vi "Exercise 4.3 Webcam to JPG.vi"() -> ()   [LabVIEW 2014]
uses:
  <vilib>/Q-Wave Systems/QwaveSys RPi Training Package (Demo)/Addons/QwaveSys RPi Training Library.lvlib
panel:
  out "Output 2":picture
  out "string":string
  in  "file path":path=path "/home/pi/temp.jpg"
  out "Output":picture
  in  "Image Size":T1(ring)
  in  "camnum":i32
  out "return type":i32
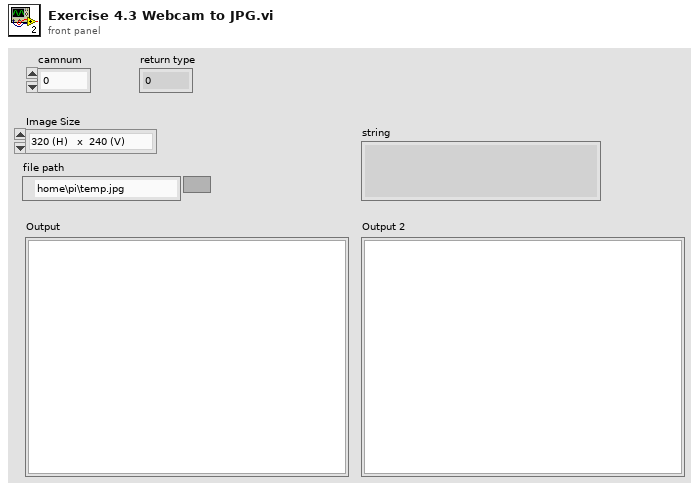
[diagram p1: front panel]
types:
  T1 = enum16{"320 (H)   x  240 (V)", "352(H)    x  288 (V)", "640 (H)   x  480 (V) ", "800 (H)   x  600 (V)", "1024 (H) x  768 (V)", "1280 (H) x  720 (V)", "1280 (H) x 1024 (V)", "1920 (H) x 1080 (V)"}
  T2 = typedef "imagedata.ctl" = cluster{"image type":i32, "image depth":i32, "image":u8[], "mask":u8[], "colors":u32[], "Rectangle":cluster{"left":i16, "top":i16, "right":i16, "bottom":i16}}
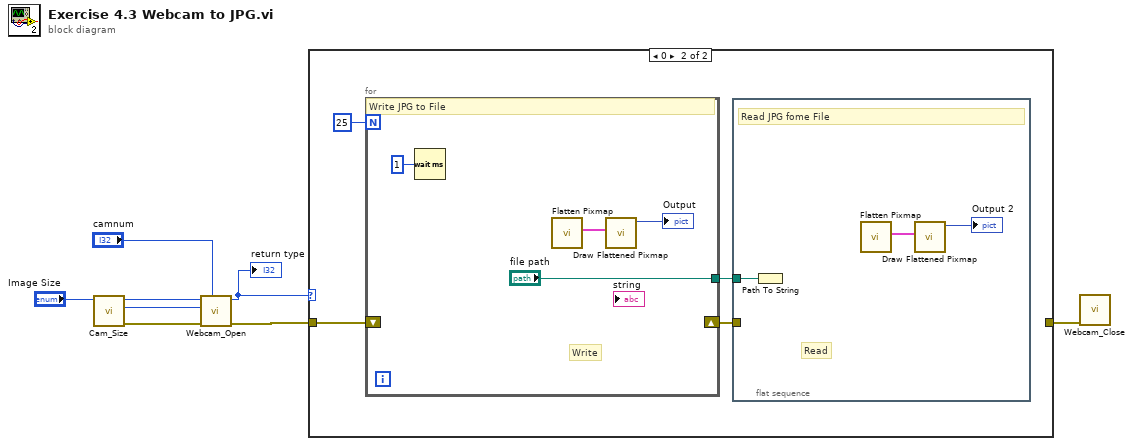
[diagram p0: block diagram]
diagram:
  n1 = call <vilib>:"Cam_Size.vi"("Image Size"="Image Size") -> ("error out"=w7:errorcluster, "h"=w6:i32, "w"=w5:i32)  [unwired: 8 in]
  n2 = call <vilib>:"Webcam_Open.vi"("webcamnum"="camnum", "error in (no error)"=w7, "height"=w6, "width"=w5) -> ("error out"=w3:errorcluster, "return type"=w2:i32)  [unwired: 6 in]
  "return type" <- w2
  n3 = case shown="0" w2 {
    tunnel: w3 -> [w9 w13]
    tunnel: [w9 _] -> w1
    frame -1, Default {
    }
    frame 0 {
      n4 = for {
        N: 25 -> [_]
        shift-right: [_] -> w10
        shift-left: w13 -> [_]
        tunnel: ["file path"] -> w11
        # "Write"
        # "Write JPG to File"
        n5 = Wait (ms)(milliseconds to wait=u32 1) -> ()  [unwired: 1 out]
        n6 = call <vilib>:"Flatten Pixmap.vi"() -> ("image data"=w19:T2)  [unwired: 11 in]
        n7 = call <vilib>:"Draw Flattened Pixmap.vi"("image data"=w19) -> ("new picture"=→"Output":picture)  [unwired: 8 in]
      }
      n8 = flat-sequence {
        tunnel: w11 -> [w16]
        tunnel: w10 -> [_]
        frame #0 {
          # "Read"
          # "Read JPG fome File"
          n9 = Path To String(path=w16) -> ()  [unwired: 1 out]
          n10 = call <vilib>:"Flatten Pixmap.vi"() -> ("image data"=w14:T2)  [unwired: 11 in]
          n11 = call <vilib>:"Draw Flattened Pixmap.vi"("image data"=w14) -> ("new picture"=→"Output 2":picture)  [unwired: 8 in]
        }
      }
    }
  }
  n12 = call <vilib>:"Webcam_Close.vi"("error in (no error)"=w1) -> ()  [unwired: 10 in, 1 out]
